vi "Set Channel Range.vi"(6 "Center (in actual channel unit)":dbl, 8 "error in (no error)":errorcluster, 9 "Channel range (in actual channel unit)":dbl, 10 "Channel":u16(ring) items=["A1"=0, "A2"=1, "A3"=2, "A4"=3, "A5"=4, "A6"=5, "A7"=6, "A8"=7, "A9"=8, "A10"=9, "K1"=200, "K2"=201, "K3"=202, "K4"=203, "FA1"=204, "FA2"=205, "FA3"=206, "FA4"=207], 11 "VISA resource name":refnum<visa-resource-name>) -> (0 "error out":errorcluster, 3 "VISA resource name out":refnum<visa-resource-name>)   [LabVIEW 2017, in "Sefram DAS220.lvlib"]
doc: "Change the channel range (according to the current channel unit).\nExample :\nTo obtain +/-5V : <B>range</B> 10V and <B>center</B> at 0V"
uses:
  <instrlib>/Sefram DAS220/Sefram DAS220.lvlib
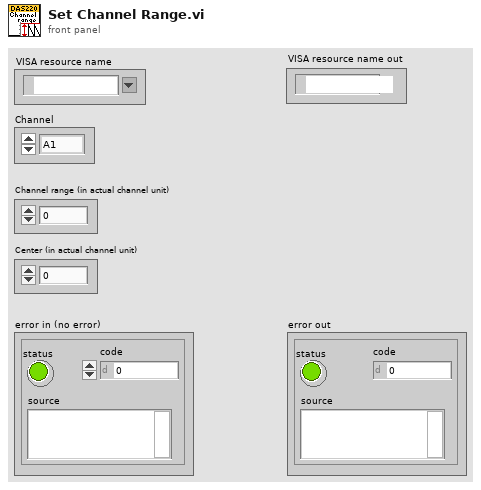
[diagram p1: front panel]
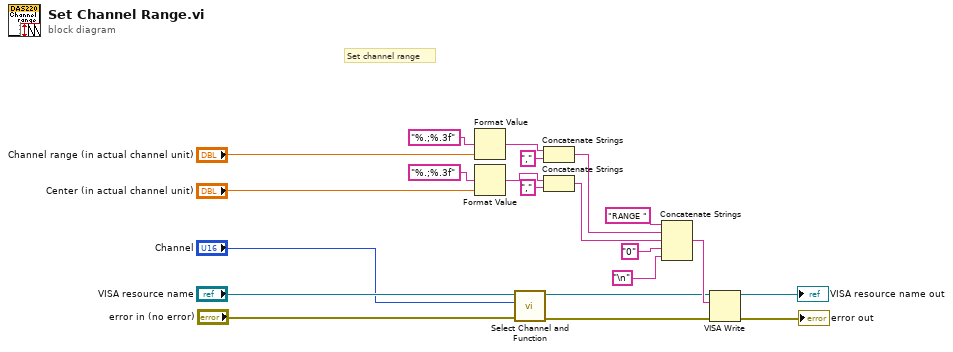
[diagram p0: block diagram]
diagram:
  # "Set channel range"
  n1 = Format Value(format string="%.;%.3f", value (0)="Channel range (in actual channel unit)") -> (output string=w7:string)  [unwired: 1 in]
  n2 = Format Value(format string="%.;%.3f", value (0)="Center (in actual channel unit)") -> (output string=w6:string)  [unwired: 1 in]
  n3 = call <instrlib>:"Select Channel and Function.vi"("error in (no error)"="error in (no error)", "Channel"="Channel", "VISA resource name"="VISA resource name") -> ("error out"=w5:errorcluster, "VISA resource name out"=w4:refnum<visa-resource-name>)  [unwired: 7 in]
  n4 = Concatenate Strings(w7, "," ("string")) -> (w17:string)
  n5 = Concatenate Strings(w6, "," ("string")) -> (w15:string)
  n6 = Concatenate Strings("RANGE " ("string"), w17, w15, "0" ("string"), "\n") -> (w21:string)
  n7 = VISA Write(VISA resource name=w4, write buffer=w21, error in (no error)=w5) -> (VISA resource name out=→"VISA resource name out":refnum<visa-resource-name>, error out=→"error out":errorcluster)  [unwired: 1 out]
